vi "Operate.vi"(8 "Error In":errorcluster, 11 "Multiply In":refnum<class "Multiply.lvclass">) -> (0 "Error Out":errorcluster, 2 "C":dbl, 3 "Multiply Out":refnum<class "Multiply.lvclass">)   [LabVIEW 2021, in "Calculator.lvlib" / "Multiply.lvclass"]
doc: "This VI is an overriding method which performs the multiplication operation."
uses:
  Multiply.lvclass
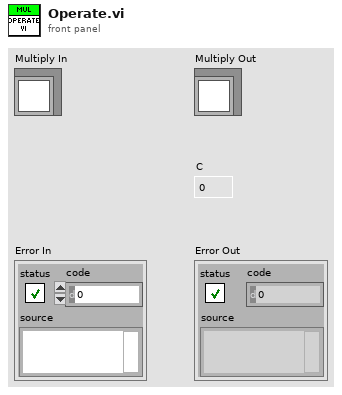
[diagram p1: front panel]
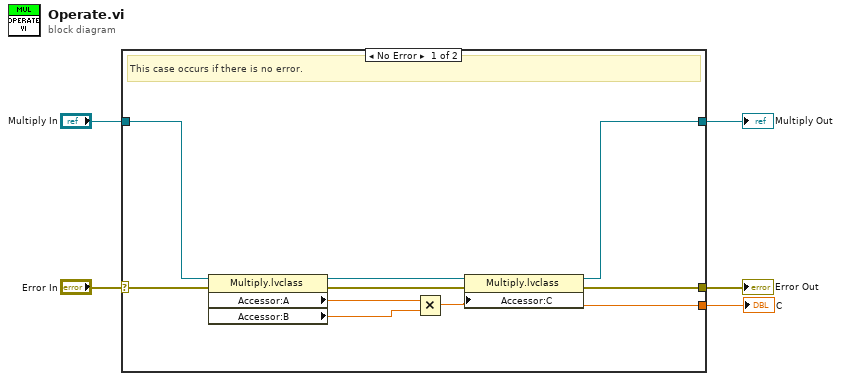
[diagram p0: block diagram]
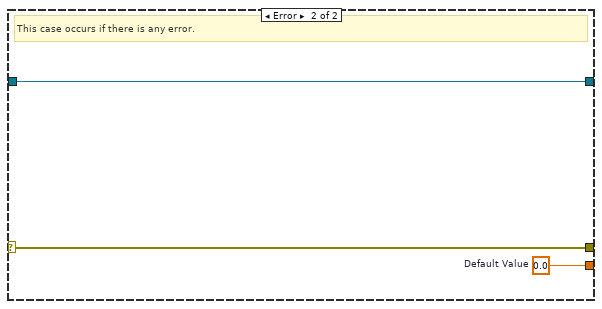
[diagram p2: hidden frame]
diagram:
  n1 = case shown="No Error" "Error In" {
    selector: "Error In" -> [w14 w16]
    tunnel: [w10 w16] -> w4
    tunnel: [w8 w15] -> w2
    tunnel: "Multiply In" -> [w7 w15]
    tunnel: [w6 w17] -> w1
    frame No Error {
      # "This case occurs if there is no error."
      n2 = property class="Multiply.lvclass"(reference=w7, error in=w14) -> (reference out=w9:refnum<class "Multiply.lvclass">, error out=w13:errorcluster, "Accessor:A"=w12:dbl, "Accessor:B"=w11:dbl)
      n3 = Multiply(x=w12, y=w11) -> (x*y=w6:dbl)
      n4 = property class="Multiply.lvclass"(reference=w9, error in=w13, "Accessor:C"=w6) -> (reference out=w8:refnum<class "Multiply.lvclass">, error out=w10:errorcluster)
    }
    frame Error {
      w17 = 0.0  # Default Value
      # "This case occurs if there is any error."
    }
  }
  "Error Out" <- w4
  "Multiply Out" <- w2
  "C" <- w1
